vi "Get DataType.vi"(8 "error in":errorcluster, 11 "DOMAIN in":refnum<class "DOMAIN.lvclass">) -> (0 "error out":errorcluster, 1 "Set?":bool, 2 "DataType":u16(ring) items=["UNKNOWN", "BOOLEAN", "INTEGER8", "INTEGER16", "INTEGER32", "UNSIGNED8", "UNSIGNED16", "UNSIGNED32", "REAL32", "VISIBLE_STRING", "OCTET_STRING", "UNICODE_STRING", "TIME_OF_DAY", "TIME_DIFFERENCE", "RESERVED1", "DOMAIN", "INTEGER24", "REAL64", "INTEGER40", "INTEGER48", "INTEGER56", "INTEGER64", "UNSIGNED24", "RESERVED2", "UNSIGNED40", "UNSIGNED48", "UNSIGNED56", "UNSIGNED64", "RESERVED3", "RESERVED4", "RESERVED5", "RESERVED6", "PDO_COMMUNICATION_PARAMETER", "PDO_MAPPING", "SDO_PARAMETER", "IDENTITY", "RESERVED7"], 3 "DOMAIN out":refnum<class "DOMAIN.lvclass">)   [LabVIEW 2019, in "Electronic Datasheet.lvlib" / "DOMAIN.lvclass"]
uses:
  DOMAIN.lvclass
  Object Type/Object Type Base.lvclass
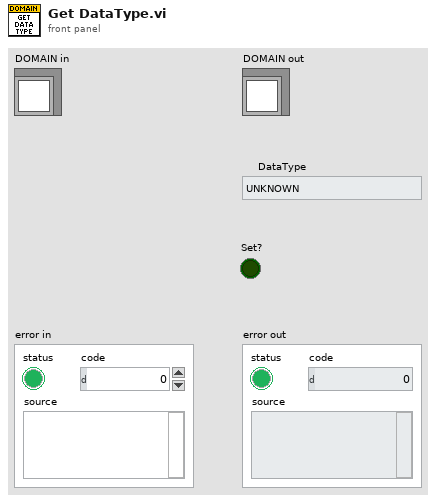
[diagram p1: front panel]
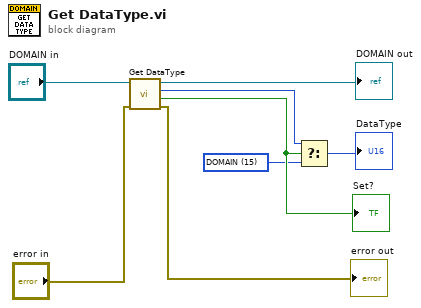
[diagram p0: block diagram]
diagram:
  w2 = u16 15 items=["UNKNOWN", "BOOLEAN", "INTEGER8", "INTEGER16", "INTEGER32", "UNSIGNED8", "UNSIGNED16", "UNSIGNED32", "REAL32", "VISIBLE_STRING", "OCTET_STRING", "UNICODE_STRING", "TIME_OF_DAY", "TIME_DIFFERENCE", "RESERVED1", "DOMAIN", "INTEGER24", "REAL64", "INTEGER40", "INTEGER48", "INTEGER56", "INTEGER64", "UNSIGNED24", "RESERVED2", "UNSIGNED40", "UNSIGNED48", "UNSIGNED56", "UNSIGNED64", "RESERVED3", "RESERVED4", "RESERVED5", "RESERVED6", "PDO_COMMUNICATION_PARAMETER", "PDO_MAPPING", "SDO_PARAMETER", "IDENTITY", "RESERVED7"] ("f")
  n1 = call-parent "Get DataType.vi"("error in"="error in", "Object Type in"="DOMAIN in") -> ("error out"=→"error out":errorcluster, "Set?"=w4:bool, "DataType"=w3:u16, "Object Type out"=→"DOMAIN out":refnum<class "DOMAIN.lvclass">)  [unwired: 6 in]
  "Set?" <- w4
  n2 = Select(t=w3, s=w4, f=w2) -> (s? t:f=→"DataType":u16)
